vi "Check if linker vi is under vilib.vi"(10 "Include VI.lib":bool, 11 "path":path) -> (3 "Include Info":bool)   [LabVIEW 2019, in "DependencyInspector.lvlib"]
uses:
  DependencyInspector.lvlib
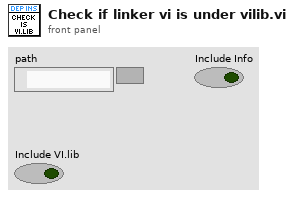
[diagram p1: front panel]
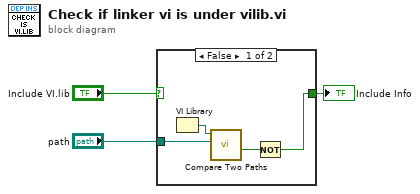
[diagram p0: block diagram]
diagram:
  n1 = case shown="False" "Include VI.lib" {
    selector: "Include VI.lib" -> [_ w8]
    tunnel: [w4 w8] -> w3
    tunnel: "path" -> [w6 _]
    frame False {
      n2 = VI Library() -> (path=w5:path)
      n3 = call <vilib>:"Compare Two Paths.vi"("Path 2"=w6, "Path 1"=w5) -> ("Path 2 Relative to Path 1?"=w7:bool)  [unwired: 6 in, 3 out]
      n4 = Not(x=w7) -> (.not. x?=w4:bool)
    }
    frame True {
    }
  }
  "Include Info" <- w3
